vi "Write PID Channels.vi"(8 "error in (no error)":errorcluster, 10 "PID Channels":T1(array[cluster]) {"output range"."output low" format="%.2f"; "output range"."output high" format="%.2f"}, 11 "Tagbus PID Module configuration in":refnum<class "Tagbus PID Module configuration.lvclass">) -> (0 "error out":errorcluster, 3 "Tagbus PID Module configuration out":refnum<class "Tagbus PID Module configuration.lvclass">)   [LabVIEW 2014, in "Tagbus PID Module configuration.lvclass"]
uses:
  Tagbus PID Module configuration.lvclass
  <vilib>/NI/Tag Bus Module Framework/channel/TBM channel.lvclass
  Tagbus PID Module configuration.lvclass/Tagbus PID Module configuration.ctl
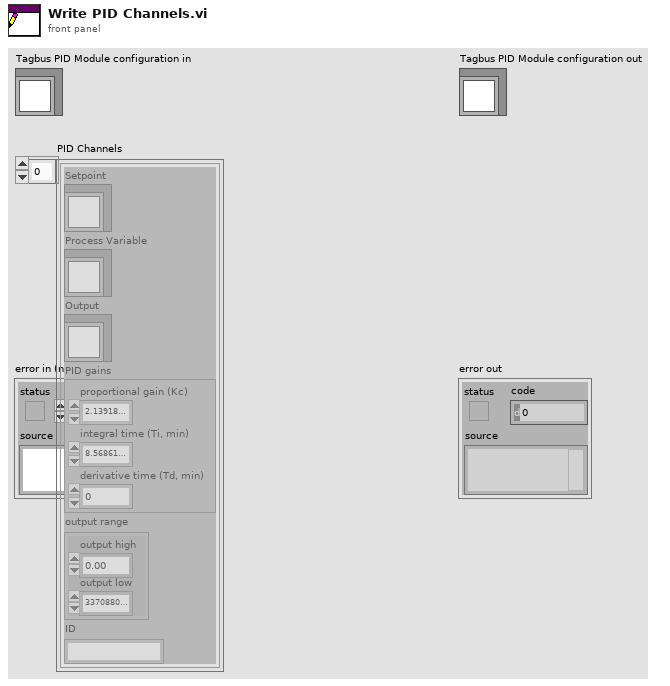
[diagram p1: front panel]
types:
  T1 = cluster{"Setpoint":refnum<class "TBM channel.lvclass">, "Process Variable":refnum<class "TBM channel.lvclass">, "Output":refnum<class "TBM channel.lvclass">, "PID gains":cluster{"proportional gain (Kc)":dbl, "integral time (Ti, min)":dbl, "derivative time (Td, min)":dbl}, "output range":cluster{"output high":dbl, "output low":dbl}, "ID":string}[]
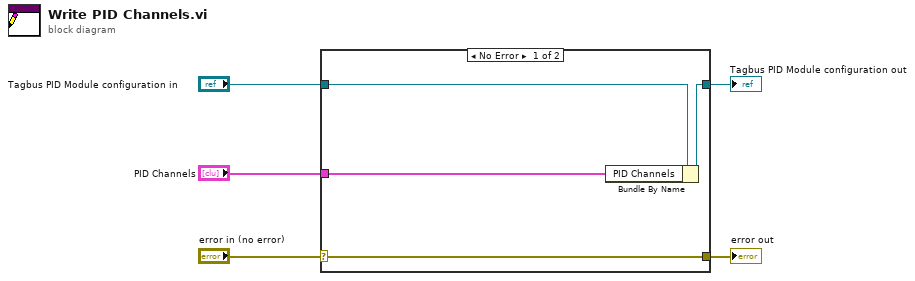
[diagram p0: block diagram]
diagram:
  n1 = case shown="No Error" "error in (no error)" {
    selector: "error in (no error)" -> [w9 w10]
    tunnel: [w9 w10] -> w4
    tunnel: [w7 w11] -> w2
    tunnel: "Tagbus PID Module configuration in" -> [w8 w11]
    tunnel: "PID Channels" -> [w6 _]
    frame No Error {
      n2 = Bundle By Name(cluster=w8, "PID Channels"=w6) -> (w7:refnum<class "Tagbus PID Module configuration.lvclass">)
    }
    frame Error {
    }
  }
  "error out" <- w4
  "Tagbus PID Module configuration out" <- w2
